vi "Digital Pattern Debugging UI.vi"() -> ()   [LabVIEW 2017, in "Engine Simulation Toolkit System Explorer.lvlib"]
uses:
  Engine Simulation Toolkit System Explorer.lvlib
  Digital Pattern.ctl
  Digital Pattern Base.ctl
  Digital Pattern Remove Edge.ctl
  Digital Pattern Add Pulse.ctl
panel:
  out "first falling":bool
  in  "get any edge":bool
  out "Any Edges":dbl[](array[numeric])
  in  "Rotations":u16=2
  out "crank angle":bool
  in  "get tooth centers":bool
  out "tooth centers":dbl[](array[numeric])
  in  "get falling":bool
  in  "get rising":bool
  out "Falling Edges":dbl[](array[numeric])
  out "Rising Edges":dbl[](array[numeric])
  out "Pattern Plot":cluster{dbl[], dbl[]}[](graph)
  in  "Zoom":cluster{dbl, dbl}(slide)={360.0, -360.0} scale=-360.0..360.0
  in  "Select Pattern":i32[](listbox)
  in  "Create Pattern":bool
  in  "Delete Pattern":bool
  in  "Down Pattern":bool
  in  "Up Pattern":bool
  in  "Edit Tab":enum32{"Blank", "Pattern"}(tab)
  in  "Base Pattern":T1
  in  "Pattern Name":string
  in  "Remove List":i32(listbox)
  in  "Add List":i32(listbox)
  in  "Remove Pulse":T2
  in  "Add Pulse":T3
  in  "Delete Pulse":bool
  in  "Create Pulse":bool
  in  "UnDelete Pulse":bool
  in  "UnCreate Pulse":bool
  in  "Cursor Tab":enum32{"Blank", "Cursor"}(tab)
  in  "Offset":sgl
  in  "Position":sgl
  in  "Tooth":i32
  in  "Merge":bool
  in  "Patterns":T4[](array[typedef])
  in  "Exit":bool
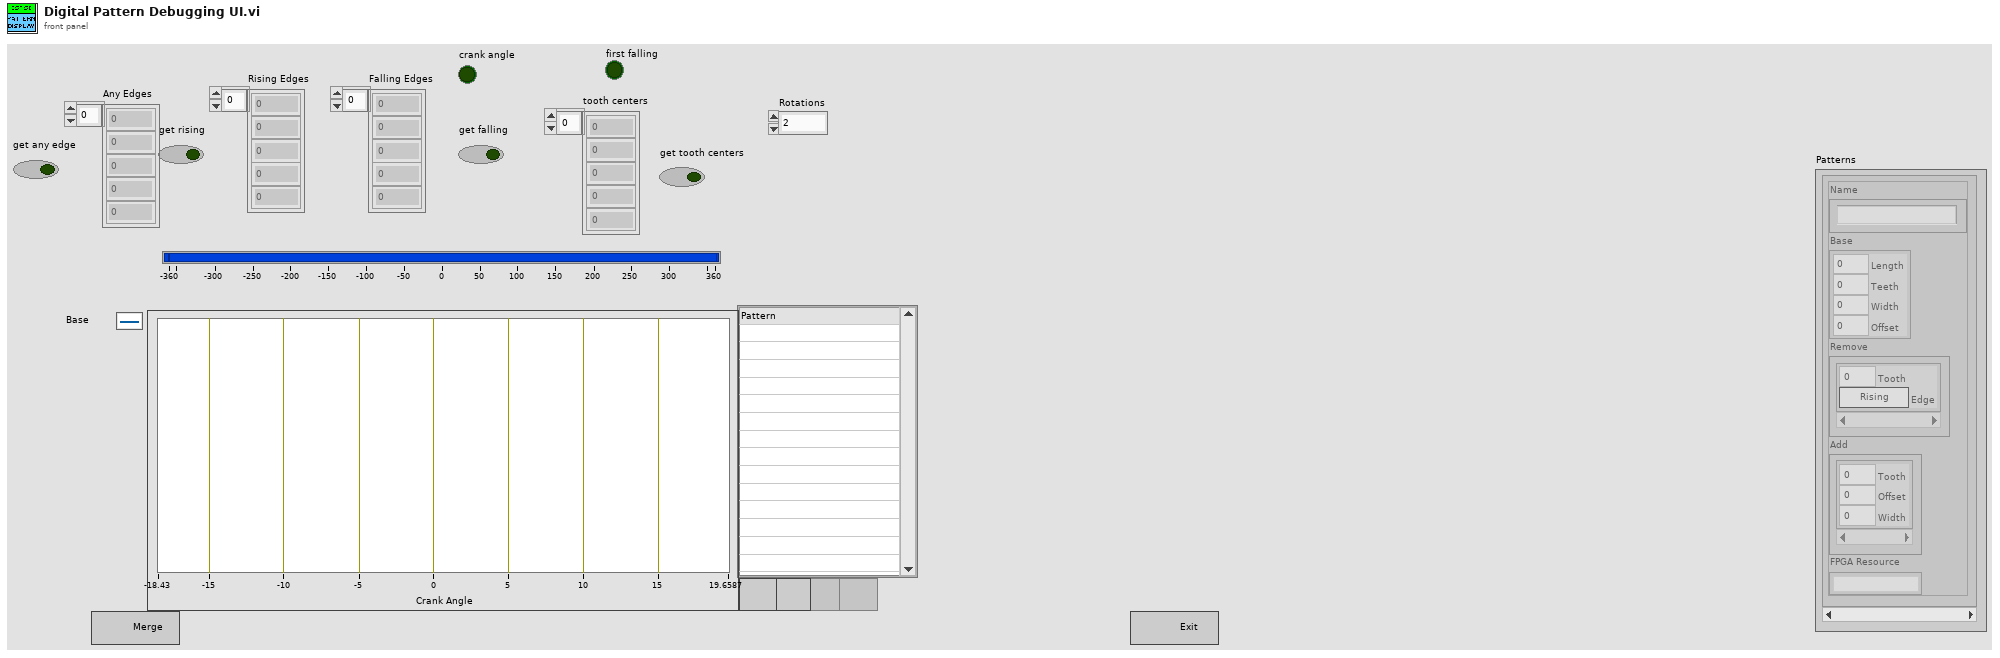
[diagram p1: front panel]
types:
  T1 = typedef "Engine Simulation Toolkit System Explorer.lvlib/Digital Pattern Base.ctl" = cluster{"Length":dbl, "Teeth":u16, "Width":dbl, "Offset":dbl}
  T2 = typedef "Engine Simulation Toolkit System Explorer.lvlib/Digital Pattern Remove Edge.ctl" = cluster{"Tooth":u16, "Edge":bool}
  T3 = typedef "Engine Simulation Toolkit System Explorer.lvlib/Digital Pattern Add Pulse.ctl" = cluster{"Tooth":u16, "Offset":dbl, "Width":dbl}
  T4 = typedef "Engine Simulation Toolkit System Explorer.lvlib/Digital Pattern.ctl" = cluster{"Name":string, "Base":T1, "Remove":T2[], "Add":T3[], "FPGA Resource":string}
  T5 = cluster{"Name":string, "Color":u32, "Style":u8, "Point Style":u8, "Name Visible":bool, "Allow Drag":bool, "Cursor Mode":u32, "Plot":i32, "Index":i32, "Position":cluster{"X":dbl, "Y":dbl}, "X Scale":u32, "Y Scale":u32, "Watch Plots":i32[], "Watch All Plots":bool, "Plot Area":i32, "Label Offset":cluster{"X":dbl, "Y":dbl}}[]
  T6 = enum8{"Enabled", "Disabled", "Disabled and Grayed Out"}
  T7 = typedef "Engine Simulation Toolkit System Explorer.lvlib/Digital Pattern Expanded.ctl" = cluster{"X":dbl[], "Y":dbl[]}
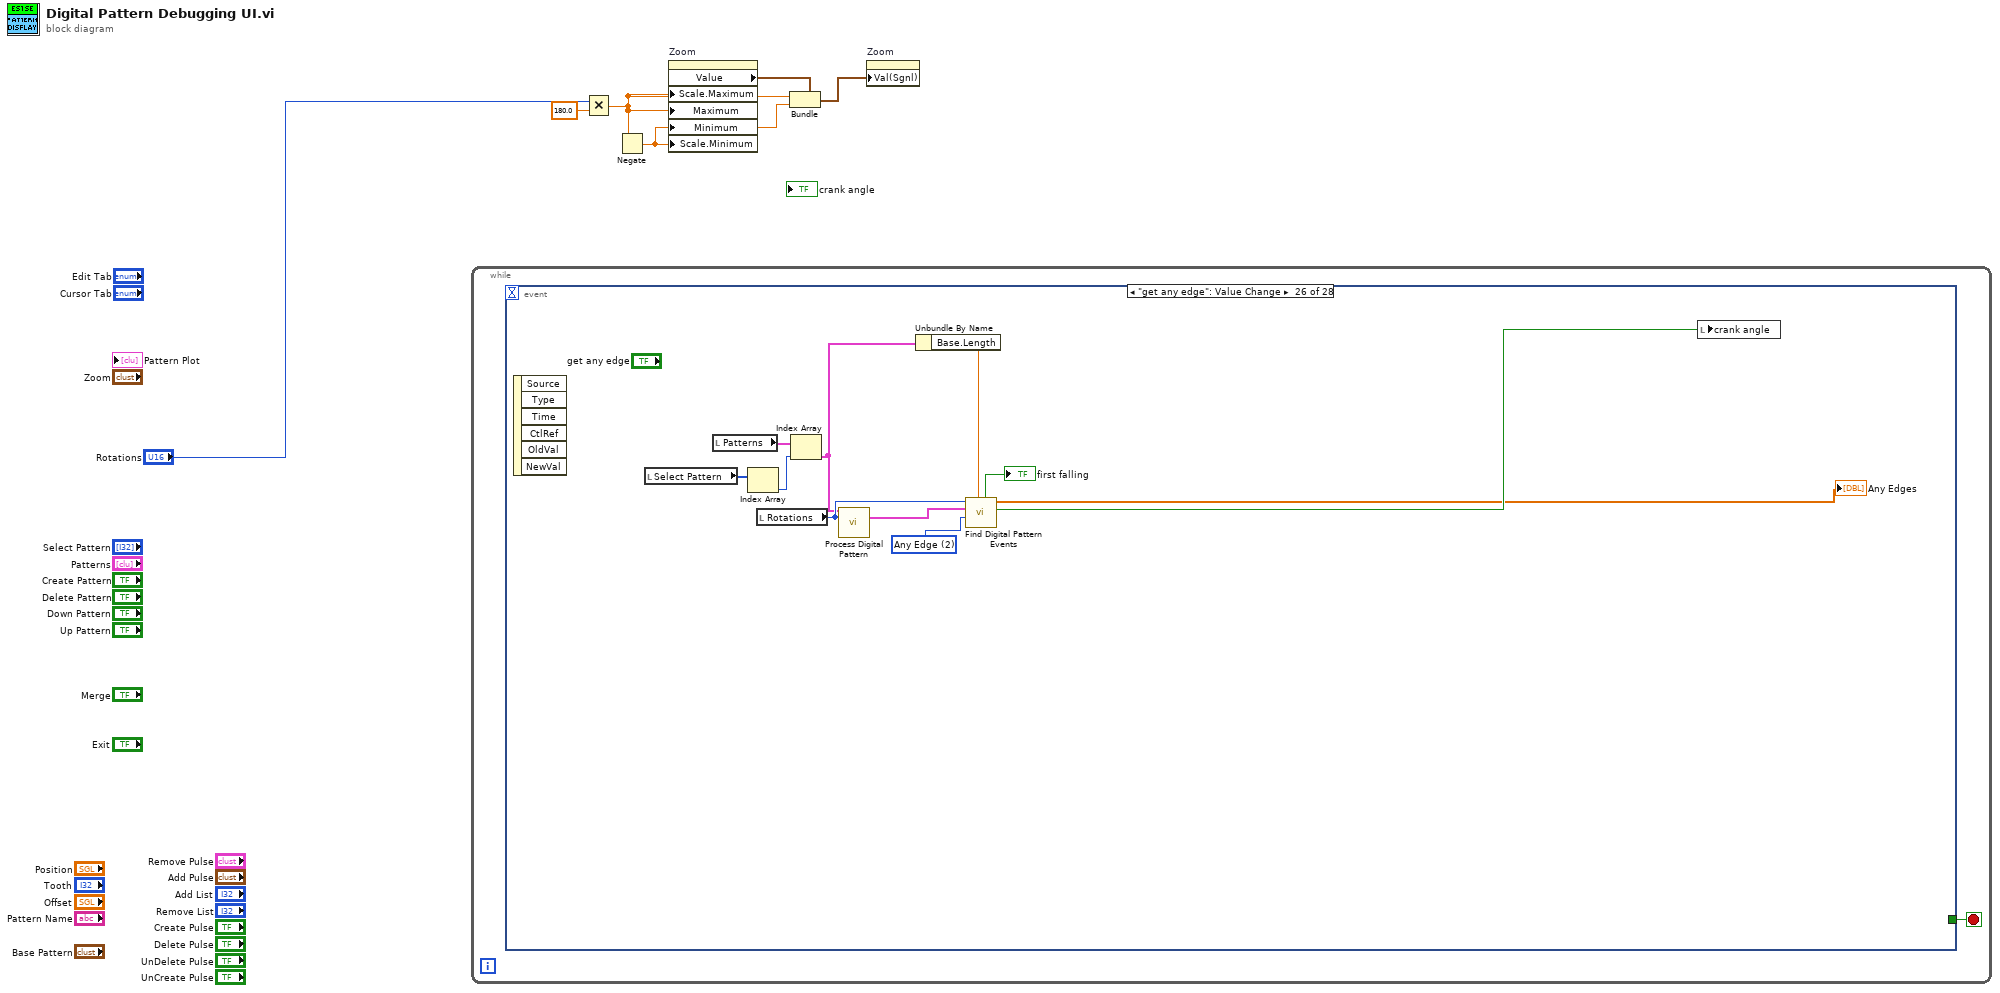
[diagram p0: block diagram]
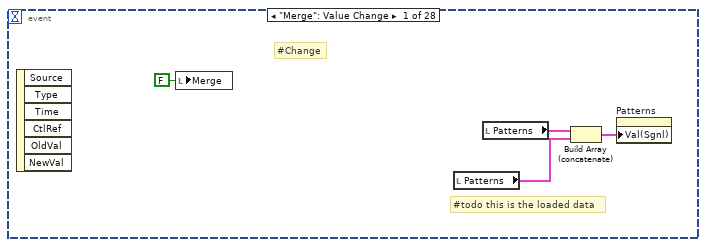
[diagram p2: hidden frame]
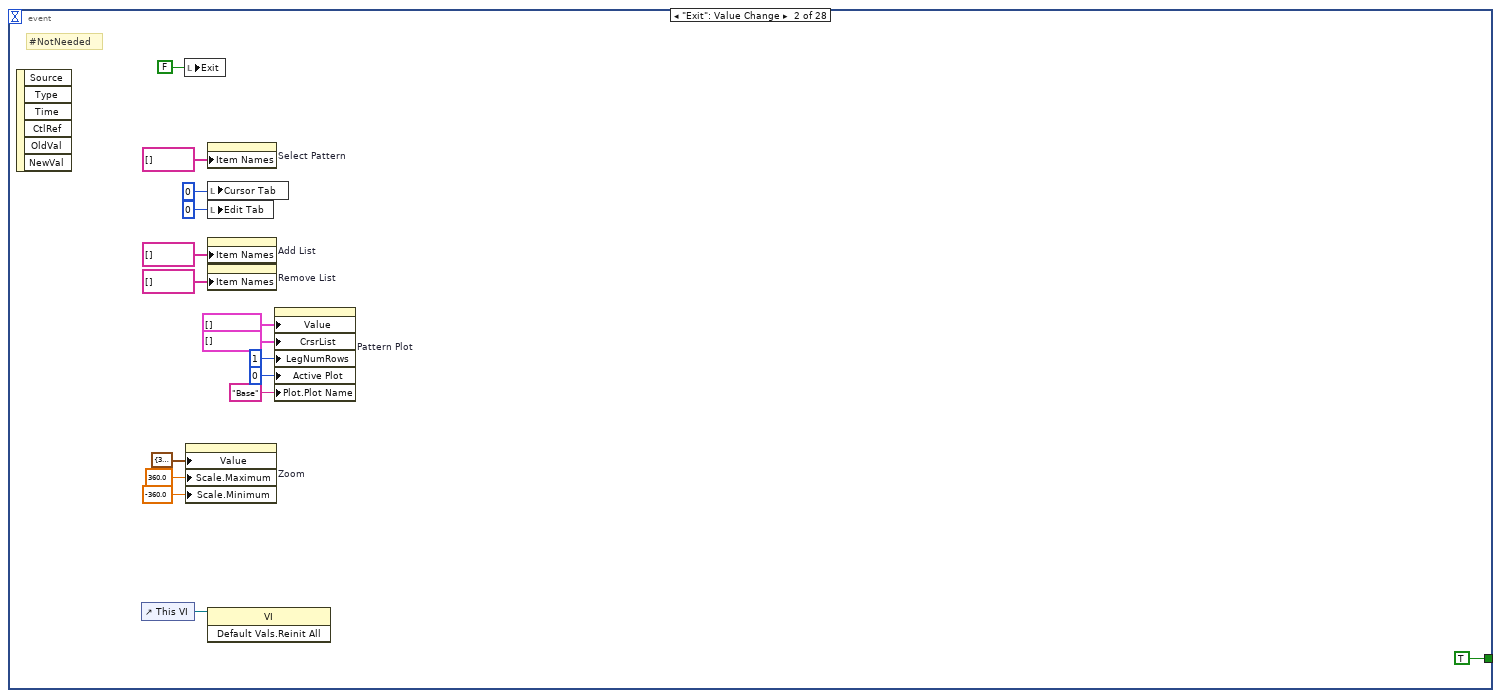
[diagram p3: hidden frame]
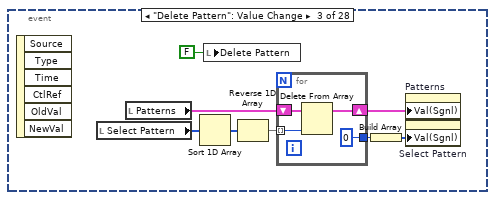
[diagram p4: hidden frame]
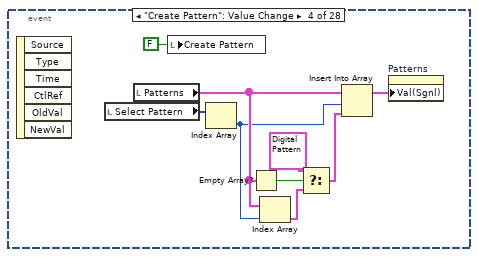
[diagram p5: hidden frame]
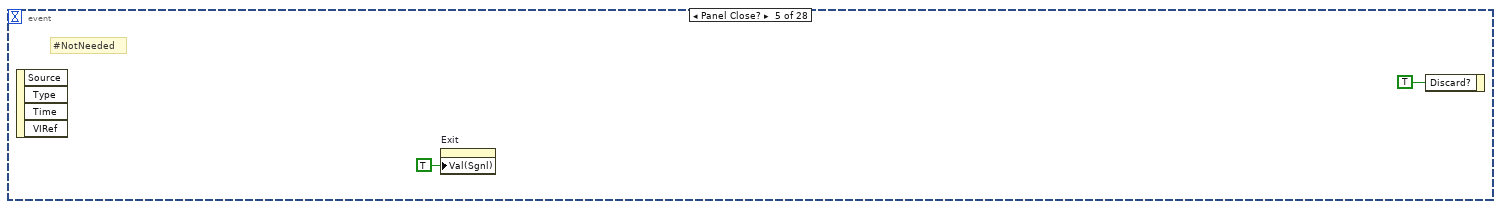
[diagram p6: hidden frame]
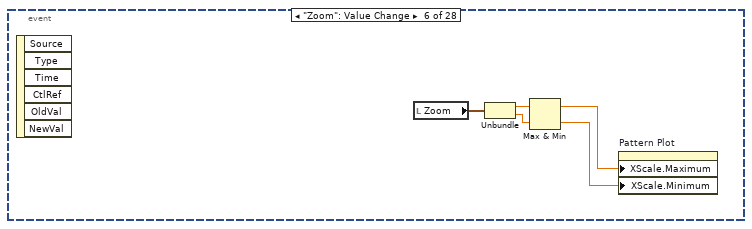
[diagram p7: hidden frame]
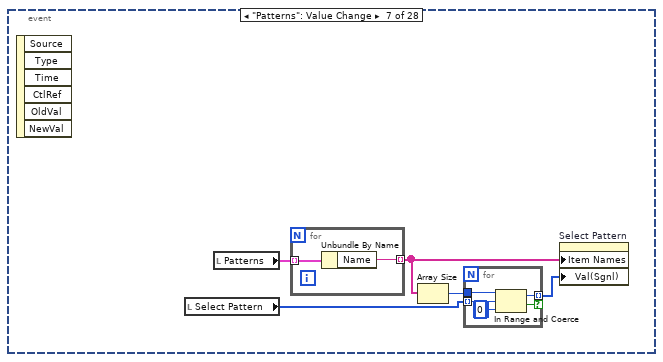
[diagram p8: hidden frame]
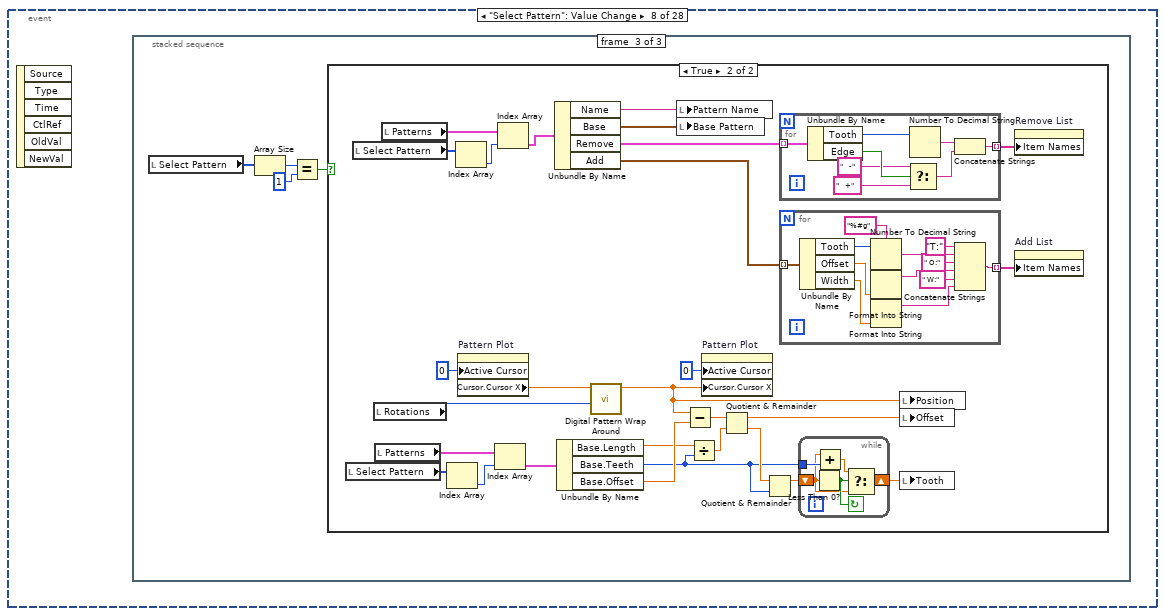
[diagram p9: hidden frame]
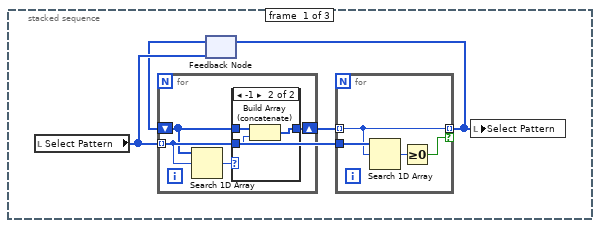
[diagram p10: hidden frame]
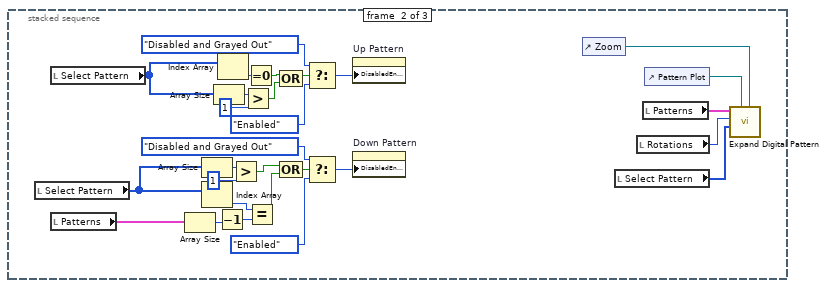
[diagram p12: hidden frame]
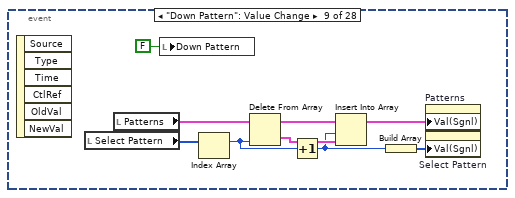
[diagram p14: hidden frame]
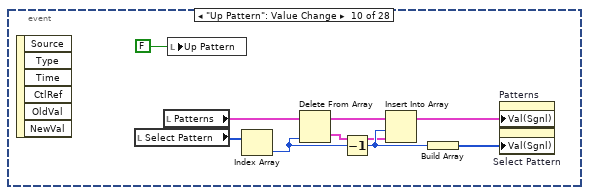
[diagram p15: hidden frame]
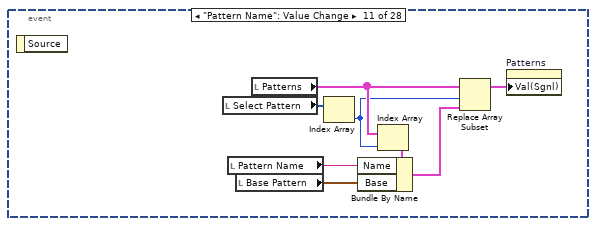
[diagram p16: hidden frame]
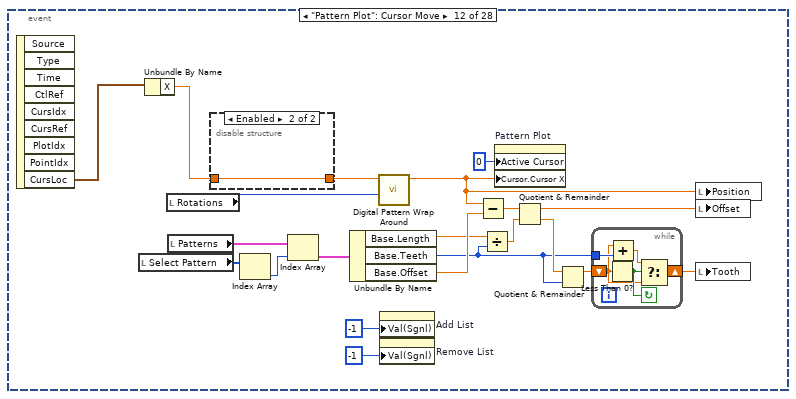
[diagram p17: hidden frame]
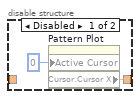
[diagram p18: hidden frame]
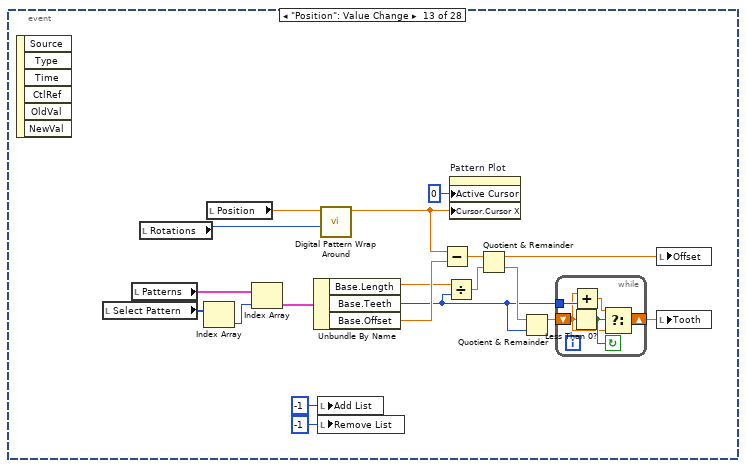
[diagram p19: hidden frame]
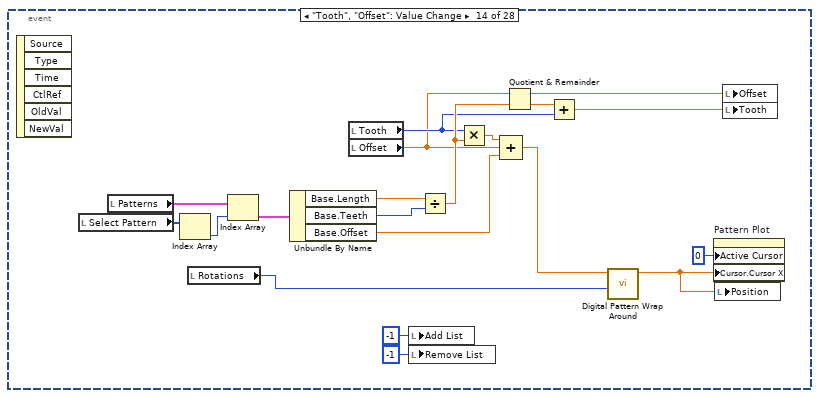
[diagram p20: hidden frame]
diagram:
  n1 = while {
    stop <- w7 stop-if-true
    n2 = event shown="[25] \"get any edge\": Value Change" {
      selector: _ -> [_ _ _ _ _ _ _ _ _ _ _ _ _ _ _ _ _ _ _ _ _ _ _ _ _ _ _ _]
      dyn-events: _ -> [_ _ _ _ _ _ _ _ _ _ _ _ _ _ _ _ _ _ _ _ _ _ _ _ _ _ _ _]
      timeout: _ -> [_ _ _ _ _ _ _ _ _ _ _ _ _ _ _ _ _ _ _ _ _ _ _ _ _ _ _ _]
      tunnel: [_ TRUE _ _ _ _ _ _ _ _ _ _ _ _ _ _ _ _ _ _ _ _ _ _ _ _ _ _] -> w7
      event "Merge": Value Change {
        # "#todo this is the loaded data"
        # "#Change"
        n3 = event-data() -> ()  [unwired: 1 in, 6 out]
        n4 = local write "Merge"(FALSE ("Open")) -> ()
        n5 = local read "Patterns"() -> (w8:T4[])
        n6 = local read "Patterns"() -> (w10:T4[])
        n7 = Build Array (concatenate)(w10, w8) -> (w9:T4[])
        n8 = property on="Patterns" class="Arr (strict)"("Val(Sgnl)"=w9) -> ()  [unwired: 2 in, 2 out]
      }
      event "Exit": Value Change {
        # "#NotNeeded"
        n9 = event-data() -> ()  [unwired: 1 in, 6 out]
        n10 = control-ref of="This VI"() -> (w16:refnum<vi>)
        n11 = local write "Exit"(FALSE ("Stop")) -> ()
        n12 = property on="Zoom" class="Slide (strict)"("Value"=cluster{dbl, dbl} {360.0, -360.0} ("Zoom"), "Scale.Maximum"=360.0 ("Scale.Range:Maximum"), "Scale.Minimum"=-360.0 ("Scale.Range:Minimum")) -> ()  [unwired: 2 in, 2 out]
        n13 = property on="Select Pattern" class="LstBox (strict)"("Item Names"=string[] []) -> ()  [unwired: 2 in, 2 out]
        n14 = local write "Cursor Tab"(0 ("y")) -> ()
        n15 = local write "Edit Tab"(0 ("y")) -> ()
        n16 = property on="Add List" class="LstBox (strict)"("Item Names"=string[] []) -> ()  [unwired: 2 in, 2 out]
        n17 = property on="Remove List" class="LstBox (strict)"("Item Names"=string[] []) -> ()  [unwired: 2 in, 2 out]
        n18 = invoke class="VI" method="Default Vals.Reinit All"(reference=w16) -> ()  [unwired: 2 in, 3 out]
        n19 = property on="Pattern Plot" class="XYGraph (strict)"("Value"=cluster{dbl[], dbl[]}[] [] ("Pattern Plot"), "CrsrList"=T5 [] ("Cursor List"), "LegNumRows"=u32 1 ("Legend:Number of Rows"), "Active Plot"=u32 0, "Plot.Plot Name"="Base") -> ()  [unwired: 2 in, 2 out]
      }
      event "Delete Pattern": Value Change {
        n20 = event-data() -> ()  [unwired: 1 in, 6 out]
        n21 = local read "Select Pattern"() -> (w30:i32[])
        n22 = local read "Patterns"() -> (w32:T4[])
        n23 = Sort 1D Array(array=w30) -> (sorted array=w33:i32[])
        n24 = local write "Delete Pattern"(FALSE ("Delete Pattern")) -> ()
        n25 = Reverse 1D Array(array=w33) -> (reversed array=w34:i32[])
        n26 = for {
          tunnel: w34 -> [w39] mode=indexing
          shift-right: [w38] -> w31
          shift-left: w32 -> [w37]
          tunnel: [0] -> w29
          n27 = Delete From Array(array=w37, index=w39) -> (array with subset deleted=w38:T4[])  [unwired: 1 in, 1 out]
        }
        n28 = Build Array(w29) -> (w28:i32[])
        n29 = property on="Patterns" class="Arr (strict)"("Val(Sgnl)"=w31) -> ()  [unwired: 2 in, 2 out]
        n30 = property on="Select Pattern" class="LstBox (strict)"("Val(Sgnl)"=w28) -> ()  [unwired: 2 in, 2 out]
      }
      event "Create Pattern": Value Change {
        n31 = event-data() -> ()  [unwired: 1 in, 6 out]
        n32 = local read "Select Pattern"() -> (w47:i32[])
        n33 = local read "Patterns"() -> (w42:T4[])
        n34 = local write "Create Pattern"(FALSE ("Create Pattern")) -> ()
        n35 = Index Array(array=w47) -> (element=w41:i32)  [unwired: 1 in]
        n36 = Empty Array?(array=w42) -> (empty?=w45:bool)
        n37 = Index Array(array=w42, index=w41) -> (element=w44:T4)
        n38 = Select(t=T4 {"Name"="New Pattern", "Base"={"Length"=360.0, "Teeth"=60, "Width"=1.0, "Offset"=-0.5}, "Remove"=[{"Tooth"=58, "Edge"=FALSE}, {"Tooth"=59, "Edge"=FALSE}], "Add"=[], "FPGA Resource"=""} ("s? t:f"), s=w45, f=w44) -> (s? t:f=w43:T4)
        n39 = Insert Into Array(array=w42, index=w41, new element=w43) -> (w46:T4[])
        n40 = property on="Patterns" class="Arr (strict)"("Val(Sgnl)"=w46) -> ()  [unwired: 2 in, 2 out]
      }
      event Panel Close? {
        # "#NotNeeded"
        n41 = event-data() -> ()  [unwired: 1 in, 4 out]
        n42 = property on="Exit" class="Bool (strict)"("Val(Sgnl)"=TRUE ("Value (Signaling)")) -> ()  [unwired: 2 in, 2 out]
        n43 = event-data("Discard?"=TRUE) -> ()  [unwired: 1 in, 1 out]
      }
      event "Zoom": Value Change {
        n44 = event-data() -> ()  [unwired: 1 in, 6 out]
        n45 = local read "Zoom"() -> (w53:cluster{dbl, dbl})
        n46 = Unbundle(w53) -> (w54:dbl, w55:dbl)
        n47 = Max & Min(x=w54, y=w55) -> (max(x,y)=w52:dbl, min(x,y)=w51:dbl)
        n48 = property on="Pattern Plot" class="XYGraph (strict)"("XScale.Maximum"=w52, "XScale.Minimum"=w51) -> ()  [unwired: 2 in, 2 out]
      }
      event "Patterns": Value Change {
        n49 = event-data() -> ()  [unwired: 1 in, 6 out]
        n50 = local read "Select Pattern"() -> (w60:i32[])
        n51 = local read "Patterns"() -> (w59:T4[])
        n52 = for {
          tunnel: w59 -> [w67] mode=indexing
          tunnel: [w66] -> w56 mode=indexing
          n53 = Unbundle By Name(w67) -> ("Name"=w66:string)
        }
        n54 = Array Size(array=w56) -> (size(s)=w57:i32)
        n55 = for {
          tunnel: w57 -> [w65]
          tunnel: [w63] -> w58 mode=indexing if=w61
          tunnel: w60 -> [w62] mode=indexing
          n56 = In Range and Coerce(upper limit=w65, x=w62, lower limit=0) -> (coerced(x)=w63:i32, In Range?=w61:bool)
        }
        n57 = property on="Select Pattern" class="LstBox (strict)"("Item Names"=w56, "Val(Sgnl)"=w58) -> ()  [unwired: 2 in, 2 out]
      }
      event "Select Pattern": Value Change {
        n58 = event-data() -> ()  [unwired: 1 in, 6 out]
        n59 = stacked-sequence {
          frame #0 {
            n60 = local read "Select Pattern"() -> (w71:i32[])
            n61 = feedback #1(w71) -> (w68:i32[])
            n62 = for {
              tunnel: w71 -> [w76] mode=indexing
              shift-right: [w77] -> w69
              shift-left: w68 -> [w78]
              n63 = Search 1D Array(1D array=w78, element=w76) -> (index of element=w79:i32)  [unwired: 1 in]
              n64 = case shown="-1" w79 {
                tunnel: w78 -> [w80 w83]
                tunnel: [w80 w82] -> w77
                tunnel: w76 -> [_ w81]
                frame Default {
                }
                frame -1 {
                  n65 = Build Array (concatenate)(w83, w81) -> (w82:i32[])
                }
              }
            }
            n66 = for {
              tunnel: w71 -> [w73]
              tunnel: w69 -> [w72] mode=indexing
              tunnel: [w72] -> w70 mode=indexing if=w74
              n67 = Search 1D Array(1D array=w73, element=w72) -> (index of element=w75:i32)  [unwired: 1 in]
              n68 = Greater Or Equal To 0?(x=w75) -> (x >= 0?=w74:bool)
            }
            n69 = feedback-in #1(w70) -> ()
            n70 = local write "Select Pattern"(w70) -> ()
          }
          frame #1 {
            n71 = local read "Select Pattern"() -> (w103:i32[])
            n72 = local read "Select Pattern"() -> (w95:i32[])
            n73 = local read "Patterns"() -> (w86:T4[])
            n74 = Array Size(array=w86) -> (size(s)=w85:i32)
            n75 = Array Size(array=w103) -> (size(s)=w102:i32)
            n76 = Index Array(array=w103) -> (element=w100:i32)  [unwired: 1 in]
            n77 = Array Size(array=w95) -> (size(s)=w93:i32)
            n78 = Decrement(x=w85) -> (x-1=w84:i32)
            n79 = Index Array(array=w95) -> (element=w96:i32)  [unwired: 1 in]
            n80 = Greater?(x=w102, y=1) -> (0:w105:bool)
            n81 = Greater?(x=w93, y=1) -> (0:w97:bool)
            n82 = Equal To 0?(x=w96) -> (x = 0?=w98:bool)
            n83 = Equal?(x=w100, y=w84) -> (x = y?=w106:bool)
            n84 = Compound Arithmetic op=OR(w98, w97) -> (w99:bool)
            n85 = Compound Arithmetic op=OR(w105, w106) -> (w104:bool)
            n86 = Select(t=T6."Disabled and Grayed Out" ("Disabled"), s=w99, f=T6."Enabled" ("Disabled")) -> (s? t:f=w90:T6)
            n87 = Select(t=T6."Disabled and Grayed Out" ("Disabled"), s=w104, f=T6."Enabled" ("Disabled")) -> (s? t:f=w89:T6)
            n88 = property on="Up Pattern" class="Bool (strict)"("DisabledEnum"=w90) -> ()  [unwired: 2 in, 2 out]
            n89 = property on="Down Pattern" class="Bool (strict)"("DisabledEnum"=w89) -> ()  [unwired: 2 in, 2 out]
            n90 = control-ref of="Zoom"() -> (w109:refnum<vi>)
            n91 = local read "Select Pattern"() -> (w111:i32[])
            n92 = local read "Rotations"() -> (w107:u16)
            n93 = local read "Patterns"() -> (w108:T4[])
            n94 = control-ref of="Pattern Plot"() -> (w110:refnum<vi>)
            n95 = call "Expand Digital Pattern.vi"("Zoom"=w109, "Pattern Plot"=w110, "Select Patterns"=w111, "Rotations"=w107, "Patterns"=w108) -> ()  [unwired: 6 in, 1 out]
          }
          frame #2 {
            n96 = local read "Select Pattern"() -> (w113:i32[])
            n97 = Array Size(array=w113) -> (size(s)=w115:i32)
            n98 = Equal?(x=w115, y=1) -> (x = y?=w112:bool)
            n99 = case shown="True" w112 {
              frame False {
              }
              frame True {
                n100 = local read "Select Pattern"() -> (w135:i32[])
                n101 = local read "Select Pattern"() -> (w142:i32[])
                n102 = local read "Rotations"() -> (w116:u16)
                n103 = local read "Patterns"() -> (w134:T4[])
                n104 = local read "Patterns"() -> (w143:T4[])
                n105 = Index Array(array=w135) -> (element=w136:i32)  [unwired: 1 in]
                n106 = Index Array(array=w142) -> (element=w141:i32)  [unwired: 1 in]
                n107 = property on="Pattern Plot" class="XYGraph (strict)"("Active Cursor"=u32 0) -> ("Cursor.Cursor X"=w118:dbl)  [unwired: 2 in, 2 out]
                n108 = Index Array(array=w134, index=w136) -> (element=w133:T4)
                n109 = Index Array(array=w143, index=w141) -> (element=w140:T4)
                n110 = Unbundle By Name(w140) -> ("Name"=w139:string, "Base"=w138:T1, "Remove"=w124:T2[], "Add"=w122:T3[])
                n111 = Unbundle By Name(w133) -> ("Base.Length"=w130:dbl, "Base.Teeth"=w127:u16, "Base.Offset"=w132:dbl)
                n112 = call "Digital Pattern Wrap Around.vi"("Rotations"=w116, "x"=w118) -> ("x"=w117:dbl)  [unwired: 9 in]
                n113 = local write "Pattern Name"(w139) -> ()
                n114 = local write "Base Pattern"(w138) -> ()
                n115 = Subtract(x=w117, y=w132) -> (x-y=w131:dbl)
                n116 = Divide(x=w130, y=w127) -> (x/y=w129:dbl)
                n117 = property on="Pattern Plot" class="XYGraph (strict)"("Active Cursor"=u32 0, "Cursor.Cursor X"=w117) -> ()  [unwired: 2 in, 2 out]
                n118 = Quotient & Remainder(x=w131, y=w129) -> (x-y*floor(x/y)=w120:dbl, floor(x/y)=w128:dbl)
                n119 = Quotient & Remainder(x=w128, y=w127) -> (x-y*floor(x/y)=w126:dbl)  [unwired: 1 out]
                n120 = for {
                  tunnel: w124 -> [w163] mode=indexing
                  tunnel: [w156] -> w123 mode=indexing
                  n121 = Unbundle By Name(w163) -> ("Tooth"=w162:u16, "Edge"=w160:bool)
                  n122 = Select(t="   -" ("string"), s=w160, f="   +" ("string")) -> (s? t:f=w159:string)
                  n123 = Number To Decimal String(number=w162) -> (decimal integer string=w161:string)  [unwired: 1 in]
                  n124 = Concatenate Strings(w161, w159) -> (w156:string)
                }
                n125 = for {
                  tunnel: w122 -> [w155] mode=indexing
                  tunnel: [w152] -> w121 mode=indexing
                  w145 = "%#g" ("format string")
                  n126 = Unbundle By Name(w155) -> ("Tooth"=w154:u16, "Offset"=w149:dbl, "Width"=w148:dbl)
                  n127 = Number To Decimal String(number=w154) -> (decimal integer string=w153:string)  [unwired: 1 in]
                  n128 = Format Into String(format string=w145, w149) -> (resulting string=w146:string)  [unwired: 2 in, 1 out]
                  n129 = Format Into String(format string=w145, w148) -> (resulting string=w147:string)  [unwired: 2 in, 1 out]
                  n130 = Concatenate Strings("T:" ("string"), w153, " O:" ("string"), w146, " W:" ("string"), w147) -> (w152:string)
                }
                n131 = while {
                  tunnel: w127 -> [w165]
                  shift-right: [w167] -> w119
                  shift-left: w126 -> [w164]
                  stop <- w168 continue-if-true
                  n132 = Less Than 0?(x=w164) -> (x < 0?=w168:bool)
                  n133 = Add(x=w164, y=w165) -> (x+y=w166:dbl)
                  n134 = Select(t=w166, s=w168, f=w164) -> (s? t:f=w167:dbl)
                }
                n135 = local write "Position"(w117) -> ()
                n136 = local write "Offset"(w120) -> ()
                n137 = local write "Tooth"(w119) -> ()
                n138 = property on="Remove List" class="LstBox (strict)"("Item Names"=w123) -> ()  [unwired: 2 in, 2 out]
                n139 = property on="Add List" class="LstBox (strict)"("Item Names"=w121) -> ()  [unwired: 2 in, 2 out]
              }
            }
          }
        }
      }
      event "Down Pattern": Value Change {
        n140 = event-data() -> ()  [unwired: 1 in, 6 out]
        n141 = local read "Select Pattern"() -> (w175:i32[])
        n142 = local read "Patterns"() -> (w176:T4[])
        n143 = local write "Down Pattern"(FALSE ("Create Engine")) -> ()
        n144 = Index Array(array=w175) -> (element=w170:i32)  [unwired: 1 in]
        n145 = Delete From Array(array=w176, index=w170) -> (deleted portion=w173:T4, array with subset deleted=w174:T4[])  [unwired: 1 in]
        n146 = Increment(x=w170) -> (x+1=w171:i32)
        n147 = Insert Into Array(array=w174, index=w171, new element=w173) -> (w172:T4[])
        n148 = Build Array(w171) -> (w169:i32[])
        n149 = property on="Patterns" class="Arr (strict)"("Val(Sgnl)"=w172) -> ()  [unwired: 2 in, 2 out]
        n150 = property on="Select Pattern" class="LstBox (strict)"("Val(Sgnl)"=w169) -> ()  [unwired: 2 in, 2 out]
      }
      event "Up Pattern": Value Change {
        n151 = event-data() -> ()  [unwired: 1 in, 6 out]
        n152 = local read "Select Pattern"() -> (w179:i32[])
        n153 = local read "Patterns"() -> (w178:T4[])
        n154 = local write "Up Pattern"(FALSE ("Create Engine")) -> ()
        n155 = Index Array(array=w179) -> (element=w185:i32)  [unwired: 1 in]
        n156 = Delete From Array(array=w178, index=w185) -> (deleted portion=w181:T4, array with subset deleted=w180:T4[])  [unwired: 1 in]
        n157 = Decrement(x=w185) -> (x-1=w183:i32)
        n158 = Insert Into Array(array=w180, index=w183, new element=w181) -> (w182:T4[])
        n159 = Build Array(w183) -> (w184:i32[])
        n160 = property on="Patterns" class="Arr (strict)"("Val(Sgnl)"=w182) -> ()  [unwired: 2 in, 2 out]
        n161 = property on="Select Pattern" class="LstBox (strict)"("Val(Sgnl)"=w184) -> ()  [unwired: 2 in, 2 out]
      }
      event "Pattern Name": Value Change {
        n162 = event-data() -> ()  [unwired: 1 in, 1 out]
        n163 = local read "Select Pattern"() -> (w194:i32[])
        n164 = local read "Pattern Name"() -> (w188:string)
        n165 = local read "Base Pattern"() -> (w187:T1)
        n166 = local read "Patterns"() -> (w192:T4[])
        n167 = Index Array(array=w194) -> (element=w191:i32)  [unwired: 1 in]
        n168 = Index Array(array=w192, index=w191) -> (element=w190:T4)
        n169 = Bundle By Name(cluster=w190, "Name"=w188, "Base"=w187) -> (w189:T4)
        n170 = Replace Array Subset(array=w192, new element=w189, index=w191) -> (w193:T4[])
        n171 = property on="Patterns" class="Arr (strict)"("Val(Sgnl)"=w193) -> ()  [unwired: 2 in, 2 out]
      }
      event "Pattern Plot": Cursor Move {
        n172 = event-data() -> ("CursLoc"=w198:cluster{"X":dbl, "Y":dbl})  [unwired: 1 in, 8 out]
        n173 = local read "Select Pattern"() -> (w214:i32[])
        n174 = Unbundle By Name(w198) -> ("X"=w197:dbl)
        n175 = local read "Rotations"() -> (w199:u16)
        n176 = local read "Patterns"() -> (w213:T4[])
        n177 = disable-structure shown="Enabled" {
          disable-tunnel: [w216 w218] -> w201
          disable-tunnel: w197 -> [_ w218]
          frame Disabled {
            n178 = property on="Pattern Plot" class="XYGraph (strict)"("Active Cursor"=u32 0) -> ("Cursor.Cursor X"=w216:dbl)  [unwired: 2 in, 2 out]
          }
          frame Enabled {
          }
        }
        n179 = Index Array(array=w214) -> (element=w215:i32)  [unwired: 1 in]
        n180 = Index Array(array=w213, index=w215) -> (element=w212:T4)
        n181 = Unbundle By Name(w212) -> ("Base.Length"=w209:dbl, "Base.Teeth"=w206:u16, "Base.Offset"=w211:dbl)
        n182 = call "Digital Pattern Wrap Around.vi"("Rotations"=w199, "x"=w201) -> ("x"=w200:dbl)  [unwired: 9 in]
        n183 = property on="Add List" class="LstBox (strict)"("Val(Sgnl)"=-1 ("Add List")) -> ()  [unwired: 2 in, 2 out]
        n184 = property on="Remove List" class="LstBox (strict)"("Val(Sgnl)"=-1 ("Remove List")) -> ()  [unwired: 2 in, 2 out]
        n185 = Subtract(x=w200, y=w211) -> (x-y=w210:dbl)
        n186 = Divide(x=w209, y=w206) -> (x/y=w208:dbl)
        n187 = property on="Pattern Plot" class="XYGraph (strict)"("Active Cursor"=u32 0, "Cursor.Cursor X"=w200) -> ()  [unwired: 2 in, 2 out]
        n188 = Quotient & Remainder(x=w210, y=w208) -> (x-y*floor(x/y)=w202:dbl, floor(x/y)=w207:dbl)
        n189 = Quotient & Remainder(x=w207, y=w206) -> (x-y*floor(x/y)=w205:dbl)  [unwired: 1 out]
        n190 = while {
          tunnel: w206 -> [w220]
          shift-right: [w222] -> w203
          shift-left: w205 -> [w219]
          stop <- w223 continue-if-true
          n191 = Less Than 0?(x=w219) -> (x < 0?=w223:bool)
          n192 = Add(x=w219, y=w220) -> (x+y=w221:dbl)
          n193 = Select(t=w221, s=w223, f=w219) -> (s? t:f=w222:dbl)
        }
        n194 = local write "Position"(w200) -> ()
        n195 = local write "Offset"(w202) -> ()
        n196 = local write "Tooth"(w203) -> ()
      }
      event "Position": Value Change {
        n197 = event-data() -> ()  [unwired: 1 in, 6 out]
        n198 = local read "Select Pattern"() -> (w240:i32[])
        n199 = local read "Patterns"() -> (w239:T4[])
        n200 = local read "Rotations"() -> (w226:u16)
        n201 = Index Array(array=w240) -> (element=w241:i32)  [unwired: 1 in]
        n202 = local read "Position"() -> (w228:sgl)
        n203 = Index Array(array=w239, index=w241) -> (element=w238:T4)
        n204 = Unbundle By Name(w238) -> ("Base.Length"=w235:dbl, "Base.Teeth"=w232:u16, "Base.Offset"=w237:dbl)
        n205 = local write "Add List"(-1 ("Add List")) -> ()
        n206 = local write "Remove List"(-1 ("Remove List")) -> ()
        n207 = call "Digital Pattern Wrap Around.vi"("Rotations"=w226, "x"=w228) -> ("x"=w227:dbl)  [unwired: 9 in]
        n208 = Subtract(x=w227, y=w237) -> (x-y=w236:dbl)
        n209 = Divide(x=w235, y=w232) -> (x/y=w234:dbl)
        n210 = property on="Pattern Plot" class="XYGraph (strict)"("Active Cursor"=u32 0, "Cursor.Cursor X"=w227) -> ()  [unwired: 2 in, 2 out]
        n211 = Quotient & Remainder(x=w236, y=w234) -> (x-y*floor(x/y)=w229:dbl, floor(x/y)=w233:dbl)
        n212 = Quotient & Remainder(x=w233, y=w232) -> (x-y*floor(x/y)=w231:dbl)  [unwired: 1 out]
        n213 = while {
          tunnel: w232 -> [w244]
          shift-right: [w246] -> w230
          shift-left: w231 -> [w243]
          stop <- w247 continue-if-true
          n214 = Less Than 0?(x=w243) -> (x < 0?=w247:bool)
          n215 = Add(x=w243, y=w244) -> (x+y=w245:dbl)
          n216 = Select(t=w245, s=w247, f=w243) -> (s? t:f=w246:dbl)
        }
        n217 = local write "Offset"(w229) -> ()
        n218 = local write "Tooth"(w230) -> ()
      }
      event "Tooth", "Offset": Value Change {
        n219 = event-data() -> ()  [unwired: 1 in, 6 out]
        n220 = local read "Select Pattern"() -> (w265:i32[])
        n221 = local read "Patterns"() -> (w264:T4[])
        n222 = Index Array(array=w265) -> (element=w266:i32)  [unwired: 1 in]
        n223 = local read "Rotations"() -> (w250:u16)
        n224 = Index Array(array=w264, index=w266) -> (element=w263:T4)
        n225 = Unbundle By Name(w263) -> ("Base.Length"=w262:dbl, "Base.Teeth"=w261:u16, "Base.Offset"=w259:dbl)
        n226 = local read "Tooth"() -> (w256:i32)
        n227 = local read "Offset"() -> (w255:sgl)
        n228 = local write "Add List"(-1 ("Add List")) -> ()
        n229 = local write "Remove List"(-1 ("Remove List")) -> ()
        n230 = Divide(x=w262, y=w261) -> (x/y=w258:dbl)
        n231 = Multiply(x=w256, y=w258) -> (x*y=w260:dbl)
        n232 = Compound Arithmetic op=ADD(w260, w255, w259) -> (w252:dbl)
        n233 = Quotient & Remainder(x=w255, y=w258) -> (x-y*floor(x/y)=w253:dbl, floor(x/y)=w257:dbl)
        n234 = Add(x=w257, y=w256) -> (x+y=w254:dbl)
        n235 = call "Digital Pattern Wrap Around.vi"("Rotations"=w250, "x"=w252) -> ("x"=w251:dbl)  [unwired: 9 in]
        n236 = property on="Pattern Plot" class="XYGraph (strict)"("Active Cursor"=u32 0, "Cursor.Cursor X"=w251) -> ()  [unwired: 2 in, 2 out]
        n237 = local write "Position"(w251) -> ()
        n238 = local write "Offset"(w253) -> ()
        n239 = local write "Tooth"(w254) -> ()
      }
      event "UnDelete Pulse": Value Change {
        n240 = event-data() -> ()  [unwired: 1 in, 6 out]
        n241 = local read "Select Pattern"() -> (w280:i32[])
        n242 = local read "Remove List"() -> (w269:i32)
        n243 = local read "Patterns"() -> (w278:T4[])
        n244 = local write "UnDelete Pulse"(FALSE ("Create Pattern")) -> ()
        n245 = Index Array(array=w280) -> (element=w277:i32)  [unwired: 1 in]
        n246 = Index Array(array=w278, index=w277) -> (element=w275:T4)
        n247 = Unbundle By Name(w275) -> ("Remove"=w274:T2[])
        n248 = Delete From Array(array=w274, index=w269) -> (array with subset deleted=w270:T2[])  [unwired: 1 in, 1 out]
        n249 = Array Size(array=w270) -> (size(s)=w273:i32)
        n250 = Bundle By Name(cluster=w275, "Remove"=w270) -> (w276:T4)
        n251 = Decrement(x=w273) -> (x-1=w272:i32)
        n252 = In Range and Coerce(upper limit=w272, x=w269, lower limit=-1) -> (coerced(x)=w268:i32)  [unwired: 1 out]
        n253 = Replace Array Subset(array=w278, new element=w276, index=w277) -> (w279:T4[])
        n254 = property on="Patterns" class="Arr (strict)"("Val(Sgnl)"=w279) -> ()  [unwired: 2 in, 2 out]
        n255 = property on="Remove List" class="LstBox (strict)"("Val(Sgnl)"=w268) -> ()  [unwired: 2 in, 2 out]
      }
      event "UnCreate Pulse": Value Change {
        n256 = event-data() -> ()  [unwired: 1 in, 6 out]
        n257 = local read "Select Pattern"() -> (w294:i32[])
        n258 = local read "Add List"() -> (w284:i32)
        n259 = local read "Patterns"() -> (w292:T4[])
        n260 = local write "UnCreate Pulse"(FALSE ("Create Pattern")) -> ()
        n261 = Index Array(array=w294) -> (element=w291:i32)  [unwired: 1 in]
        n262 = Index Array(array=w292, index=w291) -> (element=w289:T4)
        n263 = Unbundle By Name(w289) -> ("Add"=w288:T3[])
        n264 = Delete From Array(array=w288, index=w284) -> (array with subset deleted=w287:T3[])  [unwired: 1 in, 1 out]
        n265 = Array Size(array=w287) -> (size(s)=w286:i32)
        n266 = Bundle By Name(cluster=w289, "Add"=w287) -> (w290:T4)
        n267 = Decrement(x=w286) -> (x-1=w285:i32)
        n268 = Replace Array Subset(array=w292, new element=w290, index=w291) -> (w293:T4[])
        n269 = In Range and Coerce(upper limit=w285, x=w284, lower limit=-1) -> (coerced(x)=w282:i32)  [unwired: 1 out]
        n270 = property on="Patterns" class="Arr (strict)"("Val(Sgnl)"=w293) -> ()  [unwired: 2 in, 2 out]
        n271 = property on="Add List" class="LstBox (strict)"("Val(Sgnl)"=w282) -> ()  [unwired: 2 in, 2 out]
      }
      event "Delete Pulse": Value Change {
        n272 = event-data() -> ()  [unwired: 1 in, 6 out]
        n273 = local read "Select Pattern"() -> (w311:i32[])
        n274 = local read "Patterns"() -> (w309:T4[])
        n275 = local write "Delete Pulse"(FALSE ("Create Pattern")) -> ()
        n276 = Index Array(array=w311) -> (element=w308:i32)  [unwired: 1 in]
        n277 = Index Array(array=w309, index=w308) -> (element=w306:T4)
        n278 = Unbundle By Name(w306) -> ("Remove"=w305:T2[], "Base.Width"=w302:dbl)
        n279 = local read "Offset"() -> (w300:sgl)
        n280 = local read "Tooth"() -> (w299:i32)
        n281 = Less?(x=w302, y=w300) -> (x < y?=w301:bool)
        n282 = Bundle By Name(cluster=T2 {"Tooth"=0, "Edge"=FALSE} ("Cluster"), "Edge"=w301, "Tooth"=w299) -> (w303:T2)
        n283 = Build Array (concatenate)(w305, w303) -> (w298:T2[])
        n284 = Array Size(array=w298) -> (size(s)=w297:i32)
        n285 = Bundle By Name(cluster=w306, "Remove"=w298) -> (w307:T4)
        n286 = Decrement(x=w297) -> (x-1=w296:i32)
        n287 = property on="Remove List" class="LstBox (strict)"("Val(Sgnl)"=w296) -> ()  [unwired: 2 in, 2 out]
        n288 = Replace Array Subset(array=w309, new element=w307, index=w308) -> (w310:T4[])
        n289 = property on="Patterns" class="Arr (strict)"("Val(Sgnl)"=w310) -> ()  [unwired: 2 in, 2 out]
      }
      event "Create Pulse": Value Change {
        n290 = event-data() -> ()  [unwired: 1 in, 6 out]
        n291 = local read "Select Pattern"() -> (w327:i32[])
        n292 = local read "Patterns"() -> (w325:T4[])
        n293 = local write "Create Pulse"(FALSE ("Create Pattern")) -> ()
        n294 = Index Array(array=w327) -> (element=w324:i32)  [unwired: 1 in]
        n295 = Index Array(array=w325, index=w324) -> (element=w322:T4)
        n296 = Unbundle By Name(w322) -> ("Add"=w321:T3[], "Base.Width"=w318:dbl)
        n297 = local read "Offset"() -> (w316:sgl)
        n298 = local read "Tooth"() -> (w317:i32)
        n299 = Bundle By Name(cluster=T3 {"Tooth"=0, "Offset"=0.0, "Width"=0.0} ("Cluster"), "Width"=w318, "Offset"=w316, "Tooth"=w317) -> (w320:T3)
        n300 = Build Array (concatenate)(w321, w320) -> (w315:T3[])
        n301 = Array Size(array=w315) -> (size(s)=w314:i32)
        n302 = Decrement(x=w314) -> (x-1=w313:i32)
        n303 = Bundle By Name(cluster=w322, "Add"=w315) -> (w323:T4)
        n304 = property on="Add List" class="LstBox (strict)"("Val(Sgnl)"=w313) -> ()  [unwired: 2 in, 2 out]
        n305 = Replace Array Subset(array=w325, new element=w323, index=w324) -> (w326:T4[])
        n306 = property on="Patterns" class="Arr (strict)"("Val(Sgnl)"=w326) -> ()  [unwired: 2 in, 2 out]
      }
      event "Remove List": Value Change {
        n307 = event-data() -> ()  [unwired: 1 in, 6 out]
        n308 = local read "Remove List"() -> (w329:i32)
        n309 = case shown="Default" w329 {
          selector: w329 -> [_ w341]
          frame -1 {
            n310 = property on="UnDelete Pulse" class="Bool (strict)"("DisabledEnum"=T6."Disabled and Grayed Out" ("Disabled")) -> ()  [unwired: 2 in, 2 out]
            n311 = property on="Delete Pulse" class="Bool (strict)"("DisabledEnum"=T6."Enabled" ("Disabled")) -> ()  [unwired: 2 in, 2 out]
            n312 = property on="Remove Pulse" class="Clust (strict)"("DisabledEnum"=T6."Disabled and Grayed Out" ("Disabled")) -> ()  [unwired: 2 in, 2 out]
          }
          frame Default {
            n313 = local read "Select Pattern"() -> (w364:i32[])
            n314 = local read "Patterns"() -> (w363:T4[])
            n315 = property on="Add List" class="LstBox (strict)"("Val(Sgnl)"=-1 ("Value (Signaling)")) -> ()  [unwired: 2 in, 2 out]
            n316 = Index Array(array=w364) -> (element=w362:i32)  [unwired: 1 in]
            n317 = Index Array(array=w363, index=w362) -> (element=w361:T4)
            n318 = property on="UnDelete Pulse" class="Bool (strict)"("DisabledEnum"=T6."Enabled" ("Disabled")) -> ()  [unwired: 2 in, 2 out]
            n319 = property on="Delete Pulse" class="Bool (strict)"("DisabledEnum"=T6."Disabled and Grayed Out" ("Disabled")) -> ()  [unwired: 2 in, 2 out]
            n320 = local read "Select Pattern"() -> (w354:i32[])
            n321 = Unbundle By Name(w361) -> ("Base.Width"=w358:dbl, "Remove"=w360:T2[])
            n322 = local read "Patterns"() -> (w353:T4[])
            n323 = Index Array(array=w354) -> (element=w355:i32)  [unwired: 1 in]
            n324 = local read "Rotations"() -> (w333:u16)
            n325 = Index Array(array=w360, index=w341) -> (element=w337:T2)
            n326 = Index Array(array=w353, index=w355) -> (element=w352:T4)
            n327 = Unbundle By Name(w337) -> ("Tooth"=w343:u16, "Edge"=w359:bool)
            n328 = local write "Remove Pulse"(w337) -> ()
            n329 = Unbundle By Name(w352) -> ("Base.Length"=w351:dbl, "Base.Teeth"=w350:u16, "Base.Offset"=w348:dbl)
            n330 = property on="Remove Pulse" class="Clust (strict)"("DisabledEnum"=T6."Enabled" ("Disabled")) -> ()  [unwired: 2 in, 2 out]
            n331 = Select(t=w358, s=w359, f=sgl 0.0) -> (s? t:f=w342:dbl)
            n332 = Divide(x=w351, y=w350) -> (x/y=w347:dbl)
            n333 = Multiply(x=w343, y=w347) -> (x*y=w349:dbl)
            n334 = Compound Arithmetic op=ADD(w349, w342, w348) -> (w335:dbl)
            n335 = Quotient & Remainder(x=w342, y=w347) -> (x-y*floor(x/y)=w344:dbl, floor(x/y)=w346:dbl)
            n336 = Add(x=w346, y=w343) -> (x+y=w345:dbl)
            n337 = call "Digital Pattern Wrap Around.vi"("Rotations"=w333, "x"=w335) -> ("x"=w334:dbl)  [unwired: 9 in]
            n338 = property on="Pattern Plot" class="XYGraph (strict)"("Active Cursor"=u32 0, "Cursor.Cursor X"=w334) -> ()  [unwired: 2 in, 2 out]
            n339 = local write "Position"(w334) -> ()
            n340 = local write "Offset"(w344) -> ()
            n341 = local write "Tooth"(w345) -> ()
          }
        }
      }
      event "Add List": Value Change {
        n342 = event-data() -> ()  [unwired: 1 in, 6 out]
        n343 = local read "Add List"() -> (w365:i32)
        n344 = case shown="Default" w365 {
          selector: w365 -> [_ w377]
          frame -1 {
            n345 = property on="UnCreate Pulse" class="Bool (strict)"("DisabledEnum"=T6."Disabled and Grayed Out" ("Disabled")) -> ()  [unwired: 2 in, 2 out]
            n346 = property on="Create Pulse" class="Bool (strict)"("DisabledEnum"=T6."Enabled" ("Disabled")) -> ()  [unwired: 2 in, 2 out]
            n347 = property on="Add Pulse" class="Clust (strict)"("DisabledEnum"=T6."Disabled and Grayed Out" ("Disabled")) -> ()  [unwired: 2 in, 2 out]
          }
          frame Default {
            n348 = local read "Select Pattern"() -> (w397:i32[])
            n349 = local read "Patterns"() -> (w396:T4[])
            n350 = local read "Select Pattern"() -> (w390:i32[])
            n351 = local read "Patterns"() -> (w389:T4[])
            n352 = Index Array(array=w397) -> (element=w395:i32)  [unwired: 1 in]
            n353 = Index Array(array=w396, index=w395) -> (element=w394:T4)
            n354 = Index Array(array=w390) -> (element=w391:i32)  [unwired: 1 in]
            n355 = local read "Rotations"() -> (w369:u16)
            n356 = property on="UnCreate Pulse" class="Bool (strict)"("DisabledEnum"=T6."Enabled" ("Disabled")) -> ()  [unwired: 2 in, 2 out]
            n357 = property on="Create Pulse" class="Bool (strict)"("DisabledEnum"=T6."Disabled and Grayed Out" ("Disabled")) -> ()  [unwired: 2 in, 2 out]
            n358 = property on="Add Pulse" class="Clust (strict)"("DisabledEnum"=T6."Enabled" ("Disabled")) -> ()  [unwired: 2 in, 2 out]
            n359 = Index Array(array=w389, index=w391) -> (element=w388:T4)
            n360 = Unbundle By Name(w394) -> ("Add"=w393:T3[])
            n361 = Unbundle By Name(w388) -> ("Base.Length"=w387:dbl, "Base.Teeth"=w386:u16, "Base.Offset"=w384:dbl)
            n362 = Index Array(array=w393, index=w377) -> (element=w373:T3)
            n363 = Unbundle By Name(w373) -> ("Tooth"=w379:u16, "Offset"=w378:dbl)
            n364 = local write "Add Pulse"(w373) -> ()
            n365 = Divide(x=w387, y=w386) -> (x/y=w383:dbl)
            n366 = Multiply(x=w379, y=w383) -> (x*y=w385:dbl)
            n367 = property on="Remove List" class="LstBox (strict)"("Val(Sgnl)"=-1 ("Value (Signaling)")) -> ()  [unwired: 2 in, 2 out]
            n368 = Compound Arithmetic op=ADD(w385, w378, w384) -> (w371:dbl)
            n369 = Quotient & Remainder(x=w378, y=w383) -> (x-y*floor(x/y)=w380:dbl, floor(x/y)=w382:dbl)
            n370 = Add(x=w382, y=w379) -> (x+y=w381:dbl)
            n371 = call "Digital Pattern Wrap Around.vi"("Rotations"=w369, "x"=w371) -> ("x"=w370:dbl)  [unwired: 9 in]
            n372 = property on="Pattern Plot" class="XYGraph (strict)"("Active Cursor"=u32 0, "Cursor.Cursor X"=w370) -> ()  [unwired: 2 in, 2 out]
            n373 = local write "Position"(w370) -> ()
            n374 = local write "Offset"(w380) -> ()
            n375 = local write "Tooth"(w381) -> ()
          }
        }
      }
      event Value Change {
        n376 = event-data() -> ()  [unwired: 1 in, 6 out]
        n377 = local read "Select Pattern"() -> (w407:i32[])
        n378 = local read "Patterns"() -> (w405:T4[])
        n379 = Index Array(array=w407) -> (element=w404:i32)  [unwired: 1 in]
        n380 = Index Array(array=w405, index=w404) -> (element=w403:T4)
        n381 = local read "Remove Pulse"() -> (w399:T2)
        n382 = local read "Remove List"() -> (w398:i32)
        n383 = Unbundle By Name(w403) -> ("Remove"=w401:T2[])
        n384 = Replace Array Subset(array=w401, new element=w399, index=w398) -> (w400:T2[])
        n385 = Bundle By Name(cluster=w403, "Remove"=w400) -> (w402:T4)
        n386 = Replace Array Subset(array=w405, new element=w402, index=w404) -> (w406:T4[])
        n387 = property on="Patterns" class="Arr (strict)"("Val(Sgnl)"=w406) -> ()  [unwired: 2 in, 2 out]
        n388 = property on="Remove List" class="LstBox (strict)"("Val(Sgnl)"=w398) -> ()  [unwired: 2 in, 2 out]
      }
      event "Rotations": Value Change {
        n389 = event-data() -> ()  [unwired: 1 in, 6 out]
        n390 = local read "Rotations"() -> (w411:u16)
        n391 = Multiply(x=w411, y=180.0 ("t")) -> (x*y=w409:dbl)
        n392 = Negate(x=w409) -> (-x=w408:dbl)
        n393 = property on="Zoom" class="Slide (strict)"("Scale.Maximum"=w409, "Maximum"=w409, "Minimum"=w408, "Scale.Minimum"=w408) -> ("Value"=w412:cluster{dbl, dbl})  [unwired: 2 in, 2 out]
        n394 = Bundle(cluster=w412, w409, w408) -> (w413:cluster{dbl, dbl})
        n395 = property on="Zoom" class="Slide (strict)"("Val(Sgnl)"=w413) -> ()  [unwired: 2 in, 2 out]
      }
      event Value Change {
        n396 = event-data() -> ()  [unwired: 1 in, 6 out]
        n397 = local read "Select Pattern"() -> (w423:i32[])
        n398 = local read "Patterns"() -> (w421:T4[])
        n399 = Index Array(array=w423) -> (element=w420:i32)  [unwired: 1 in]
        n400 = Index Array(array=w421, index=w420) -> (element=w419:T4)
        n401 = local read "Add Pulse"() -> (w415:T3)
        n402 = local read "Add List"() -> (w414:i32)
        n403 = Unbundle By Name(w419) -> ("Add"=w417:T3[])
        n404 = Replace Array Subset(array=w417, new element=w415, index=w414) -> (w416:T3[])
        n405 = Bundle By Name(cluster=w419, "Add"=w416) -> (w418:T4)
        n406 = Replace Array Subset(array=w421, new element=w418, index=w420) -> (w422:T4[])
        n407 = property on="Patterns" class="Arr (strict)"("Val(Sgnl)"=w422) -> ()  [unwired: 2 in, 2 out]
        n408 = property on="Add List" class="LstBox (strict)"("Val(Sgnl)"=w414) -> ()  [unwired: 2 in, 2 out]
      }
      event "Select Pattern": Mouse Up {
        n409 = event-data() -> ()  [unwired: 1 in, 8 out]
        n410 = local read "Select Pattern"() -> (w432:i32[])
        n411 = Array Size(array=w432) -> (size(s)=w430:i32)
        n412 = Equal?(x=w430, y=1) -> (x = y?=w425:bool)
        n413 = Select(t=1 ("y"), s=w425, f=0 ("y")) -> (s? t:f=w433:i32)
        n414 = Select(t=1 ("y"), s=w425, f=0 ("y")) -> (s? t:f=w424:i32)
        n415 = local write "Edit Tab"(w433) -> ()
        n416 = local write "Cursor Tab"(w424) -> ()
      }
      event "get rising": Value Change {
        w440 = 0 items=["Rising Edge", "Falling Edge", "Any Edge", "Center Tooth", "Center Gap"] ("Sensor")
        n417 = event-data() -> ()  [unwired: 1 in, 6 out]
        n418 = local read "Select Pattern"() -> (w443:i32[])
        n419 = local read "Patterns"() -> (w442:T4[])
        n420 = Index Array(array=w443) -> (element=w441:i32)  [unwired: 1 in]
        n421 = local read "Rotations"() -> (w439:u16)
        n422 = Index Array(array=w442, index=w441) -> (element=w437:T4)
        n423 = call "Process Digital Pattern.vi"("EPT Pattern"=w437, "Rotations"=w439) -> ("Final"=w438:T7)  [unwired: 7 in, 6 out]
        n424 = Unbundle By Name(w437) -> ("Base.Length"=w436:dbl)
        n425 = call "Find Digital Pattern Events.vi"("Base.length"=w436, "Event"=w440, "Pattern"=w438, "Rotations"=w439) -> ("crank angle"=w435:bool, "Locations"=→"Rising Edges":dbl[])  [unwired: 5 in, 1 out]
        n426 = local write "crank angle"(w435) -> ()
      }
      event "get any edge": Value Change {
        w451 = 2 items=["Rising Edge", "Falling Edge", "Any Edge", "Center Tooth", "Center Gap"] ("Sensor")
        n427 = event-data() -> ()  [unwired: 1 in, 6 out]
        n428 = local read "Select Pattern"() -> (w454:i32[])
        n429 = local read "Patterns"() -> (w453:T4[])
        n430 = Index Array(array=w454) -> (element=w452:i32)  [unwired: 1 in]
        n431 = local read "Rotations"() -> (w450:u16)
        n432 = Index Array(array=w453, index=w452) -> (element=w449:T4)
        n433 = call "Process Digital Pattern.vi"("EPT Pattern"=w449, "Rotations"=w450) -> ("Reduced"=w444:T7)  [unwired: 7 in, 6 out]
        n434 = Unbundle By Name(w449) -> ("Base.Length"=w448:dbl)
        n435 = call "Find Digital Pattern Events.vi"("Base.length"=w448, "Event"=w451, "Pattern"=w444, "Rotations"=w450) -> ("crank angle"=w447:bool, "Locations"=→"Any Edges":dbl[], "first falling"=→"first falling":bool)  [unwired: 5 in]
        n436 = local write "crank angle"(w447) -> ()
      }
      event "get tooth centers": Value Change {
        w461 = 3 items=["Rising Edge", "Falling Edge", "Any Edge", "Center Tooth", "Center Gap"] ("Sensor")
        n437 = event-data() -> ()  [unwired: 1 in, 6 out]
        n438 = local read "Select Pattern"() -> (w464:i32[])
        n439 = local read "Patterns"() -> (w463:T4[])
        n440 = Index Array(array=w464) -> (element=w462:i32)  [unwired: 1 in]
        n441 = local read "Rotations"() -> (w460:u16)
        n442 = Index Array(array=w463, index=w462) -> (element=w458:T4)
        n443 = call "Process Digital Pattern.vi"("EPT Pattern"=w458, "Rotations"=w460) -> ("Final"=w459:T7)  [unwired: 7 in, 6 out]
        n444 = Unbundle By Name(w458) -> ("Base.Length"=w457:dbl)
        n445 = call "Find Digital Pattern Events.vi"("Base.length"=w457, "Event"=w461, "Pattern"=w459, "Rotations"=w460) -> ("crank angle"=w455:bool, "Locations"=→"tooth centers":dbl[])  [unwired: 5 in, 1 out]
        n446 = local write "crank angle"(w455) -> ()
      }
      event "get falling": Value Change {
        w471 = 1 items=["Rising Edge", "Falling Edge", "Any Edge", "Center Tooth", "Center Gap"] ("Sensor")
        n447 = event-data() -> ()  [unwired: 1 in, 6 out]
        n448 = local read "Select Pattern"() -> (w474:i32[])
        n449 = local read "Patterns"() -> (w473:T4[])
        n450 = Index Array(array=w474) -> (element=w472:i32)  [unwired: 1 in]
        n451 = local read "Rotations"() -> (w470:u16)
        n452 = Index Array(array=w473, index=w472) -> (element=w468:T4)
        n453 = call "Process Digital Pattern.vi"("EPT Pattern"=w468, "Rotations"=w470) -> ("Final"=w469:T7)  [unwired: 7 in, 6 out]
        n454 = Unbundle By Name(w468) -> ("Base.Length"=w467:dbl)
        n455 = call "Find Digital Pattern Events.vi"("Base.length"=w467, "Event"=w471, "Pattern"=w469, "Rotations"=w470) -> ("crank angle"=w465:bool, "Locations"=→"Falling Edges":dbl[])  [unwired: 5 in, 1 out]
        n456 = local write "crank angle"(w465) -> ()
      }
    }
  }
  n457 = Multiply(x="Rotations", y=180.0 ("t")) -> (x*y=w3:dbl)
  n458 = Negate(x=w3) -> (-x=w2:dbl)
  n459 = property on="Zoom" class="Slide (strict)"("Scale.Maximum"=w3, "Maximum"=w3, "Minimum"=w2, "Scale.Minimum"=w2) -> ("Value"=w5:cluster{dbl, dbl})  [unwired: 2 in, 2 out]
  n460 = Bundle(cluster=w5, w3, w2) -> (w4:cluster{dbl, dbl})
  n461 = property on="Zoom" class="Slide (strict)"("Val(Sgnl)"=w4) -> ()  [unwired: 2 in, 2 out]
